vi "Inter_device_post_ops.vi"(8 "error in (no error)":errorcluster, 10 "UUT index":i32, 11 "Profibus in":refnum<class "Profibus.lvclass">) -> (0 "error out":errorcluster, 3 "Profibus out":refnum<class "Profibus.lvclass">)   [LabVIEW 2016, in "Profibus.lvclass"]
doc: "Operations performed after a UUT is interrogated. For example, Profibus must be disconnected between UUT connections."
uses:
  Profibus.lvclass
  Profibus VISA Driver/DF PROFI II.llb/CS_PB_DPV1_MSAC2_AbortReqData.ctl
  Profibus.lvclass/Profibus.ctl
  Protocol Class/Protocol.lvclass
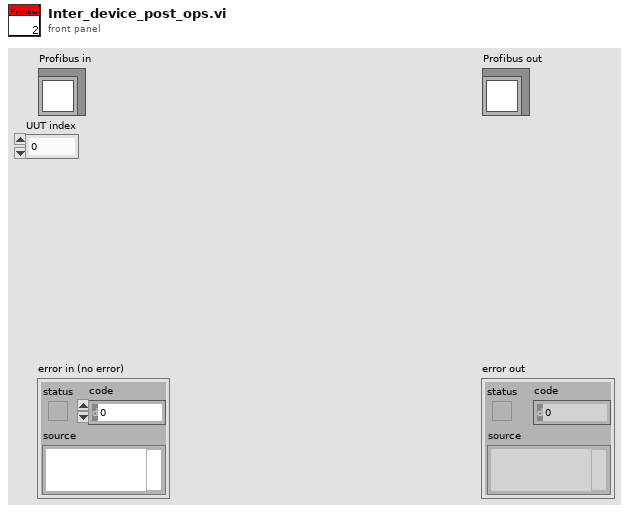
[diagram p1: front panel]
types:
  T1 = typedef "CS_PB_DPV1_MSAC2_AbortReqData.ctl" = cluster{"Communication ref.:":u8, "Subnet:":u8, "Instance &\nReasoncode:":u8, "Additional detail:":u16}
  T2 = cluster{"Device address":i32, "Switch index":i32, "Communication ref.:":u8}[]
  T3 = cluster{"Device address":i32, "Switch index":i32, "Communication ref.:":u8}
  T4 = cluster{"Error":bool, "Status":i32, "Info":string}
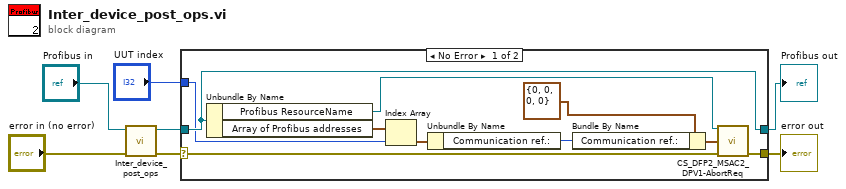
[diagram p0: block diagram]
diagram:
  n1 = call-parent "Inter_device_post_ops.vi"("error in (no error)"="error in (no error)", "Protocol in"="Profibus in") -> ("error out"=w5:errorcluster, "Protocol out"=w2:refnum<class "Profibus.lvclass">)  [unwired: 8 in]
  n2 = case shown="No Error" w5 {
    selector: w5 -> [w15 w19]
    tunnel: [w14 w19] -> w4
    tunnel: [w13 w18] -> w3
    tunnel: w2 -> [w13 w18]
    tunnel: "UUT index" -> [w11 _]
    frame No Error {
      n3 = Unbundle By Name(w13) -> ("Profibus ResourceName"=w8:refnum<visa-resource-name>, "Array of Profibus addresses"=w12:T2)
      n4 = Index Array(array=w12, index=w11) -> (element=w10:T3)
      n5 = Unbundle By Name(w10) -> ("Communication ref.:"=w9:u8)
      n6 = Bundle By Name(cluster=T1 {"Communication ref.:"=0, "Subnet:"=0, "Instance &\nReasoncode:"=0, "Additional detail:"=0} ("Abort data"), "Communication ref.:"=w9) -> (w16:T1)
      n7 = call "CS_DFP2_MSAC2_DPV1-AbortReq.vi"("DFP2 resource name"=w8, "Abort data"=w16, "Error in:"=w15) -> ("Error out:"=w14:T4)  [unwired: 9 in, 3 out]
    }
    frame Error {
    }
  }
  "error out" <- w4
  "Profibus out" <- w3
